vi "GetTextInformation.vi"(8 "error in (no error)":errorcluster, 10 "Input":string, 11 "Code128 in":refnum<class "Code128.lvclass">) -> (0 "error out":errorcluster, 1 "Text":string, 2 "Text Positions":T1[](array[typedef]), 3 "Code128 out":refnum<class "Code128.lvclass">)   [LabVIEW 2013, in "BarCodes.lvlib" / "Code128.lvclass"]
doc: "Returns an array of clusters describing how text will be sized and positioned and the actual text to place below the bar code. The Start Index is the index in the returned string that each text info entry refers to. The length is the number of characters in the returned string that each text info entry refers to. The Text Rectangle is the rectangle to draw text in. The Clearing Rectangle is the rectangle to paint with the barcode's light color to make the text clear and visible. The font information is passed into the text writing function."
uses:
  Code128.lvclass
  BarCode/TextPosition.ctl
  BarCodes.lvlib
  BarCode/BarCode.lvclass
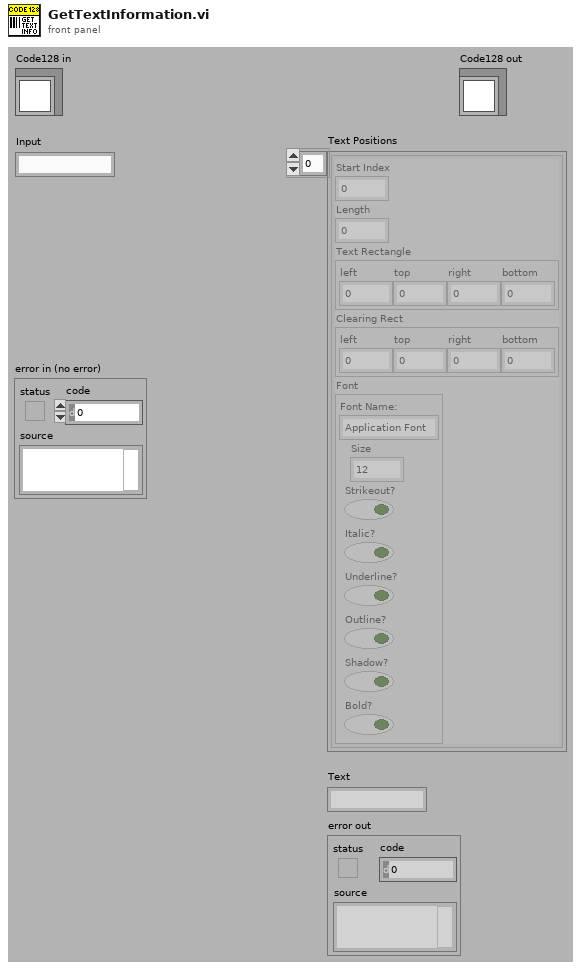
[diagram p1: front panel]
types:
  T1 = typedef "BarCodes.lvlib/BarCode.lvclass/TextPosition.ctl" = cluster{"Start Index":u8, "Length":u8, "Text Rectangle":cluster{"left":i16, "top":i16, "right":i16, "bottom":i16}, "Clearing Rect":cluster{"left":i16, "top":i16, "right":i16, "bottom":i16}, "Font":cluster{"Font Name:":string, "Size":i16, "Strikeout?":bool, "Italic?":bool, "Underline?":bool, "Outline?":bool, "Shadow?":bool, "Bold?":bool}}
  T2 = cluster{"left":i16, "top":i16, "right":i16, "bottom":i16}
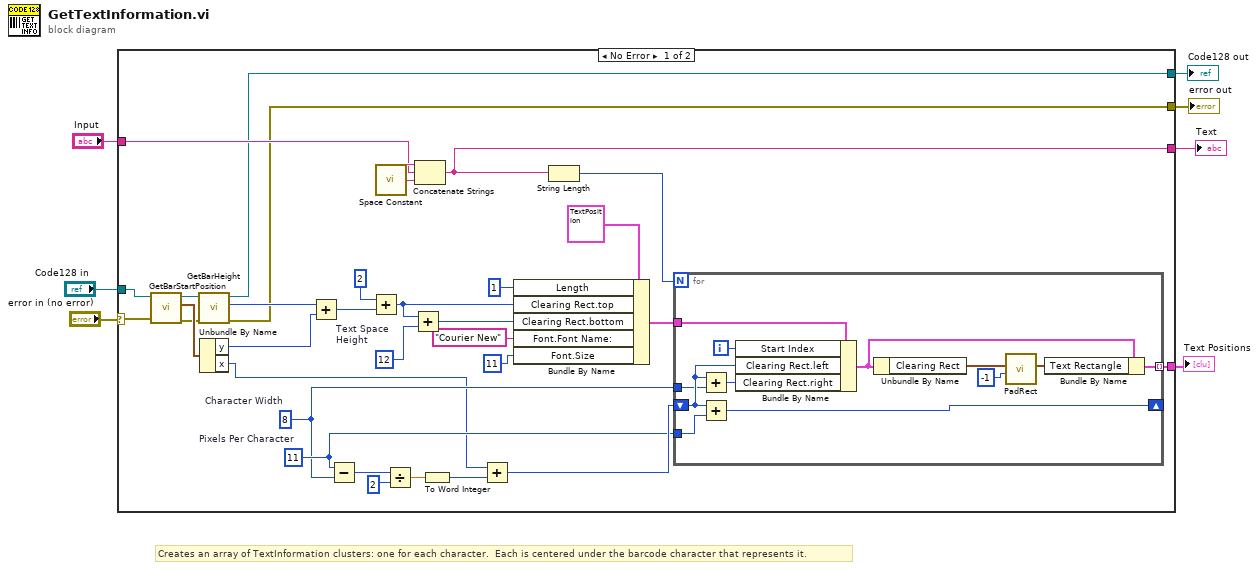
[diagram p0: block diagram]
diagram:
  # "Creates an array of TextInformation clusters: one for each character.  Each is centered under the barcode character that represents it."
  n1 = case shown="No Error" "error in (no error)" {
    selector: "error in (no error)" -> [w10 w52]
    tunnel: "Input" -> [w17 w54]
    tunnel: [w16 _] -> w6
    tunnel: [w15 w54] -> w5
    tunnel: "Code128 in" -> [w14 w53]
    tunnel: [w13 w53] -> w3
    tunnel: [w12 w52] -> w2
    frame No Error {
      w28 = i16 11  # Pixels Per Character
      w20 = i16 8  # Character Width
      w24 = i16 12  # Text Space Height
      n2 = call-dynamic "GetBarStartPosition.vi"("error in (no error)"=w10, "Code128 in"=w14) -> ("error out"=w37:errorcluster, "Start Position"=w39:cluster{"x":i16, "y":i16}, "Code128 out"=w38:refnum<class "Code128.lvclass">)  [unwired: 7 in]
      n3 = call-dynamic "GetBarHeight.vi"("error in (no error)"=w37, "Code128 in"=w38) -> ("error out"=w12:errorcluster, "Bar Height"=w36:u8, "Code128 out"=w13:refnum<class "Code128.lvclass">)  [unwired: 7 in]
      n4 = Unbundle By Name(w39) -> ("y"=w11:i16, "x"=w8:i16)
      n5 = Add(x=w36, y=w11) -> (x+y=w19:i16)
      n6 = Subtract(x=w28, y=w20) -> (x-y=w34:i16)
      n7 = Add(x=i16 2 ("y"), y=w19) -> (x+y=w18:i16)
      n8 = call <vilib>:"Space Constant.vi"() -> ("String"=w35:string)
      n9 = Divide(x=w34, y=i16 2) -> (x/y=w32:dbl)
      n10 = Add(x=w18, y=w24) -> (x+y=w23:i16)
      n11 = Concatenate Strings(w35, w17, w35) -> (w15:string)
      n12 = To Word Integer(number=w32) -> (16bit integer=w31:i16)
      n13 = Add(x=w8, y=w31) -> (x+y=w30:i16)
      n14 = Bundle By Name(cluster=T1 {"Start Index"=0, "Length"=0, "Text Rectangle"={"left"=0, "top"=0, "right"=0, "bottom"=0}, "Clearing Rect"={"left"=0, "top"=0, "right"=0, "bottom"=0}, "Font"={"Font Name:"="Application Font", "Size"=12, "Strikeout?"=FALSE, "Italic?"=FALSE, "Underline?"=FALSE, "Outline?"=FALSE, "Shadow?"=FALSE, "Bold?"=FALSE}} ("Text Position"), "Length"=u8 1, "Clearing Rect.top"=w18, "Clearing Rect.bottom"=w23, "Font.Font Name:"="Courier New", "Font.Size"=i16 11) -> (w21:T1)
      n15 = String Length(string=w15) -> (length=w29:i32)
      n16 = for {
        N: w29 -> [_]
        tunnel: w28 -> [w43]
        shift-right: [w41] -> _
        shift-left: w30 -> [w44]
        tunnel: w21 -> [w51]
        tunnel: [w46] -> w16 mode=indexing
        tunnel: w20 -> [w42]
        i -> [w40]
        n17 = Add(x=w44, y=w42) -> (x+y=w45:i16)
        n18 = Add(x=w44, y=w43) -> (x+y=w41:i16)
        n19 = Bundle By Name(cluster=w51, "Start Index"=w40, "Clearing Rect.left"=w44, "Clearing Rect.right"=w45) -> (w47:T1)
        n20 = Unbundle By Name(w47) -> ("Clearing Rect"=w50:T2)
        n21 = call "PadRect.vi"("Padding"=i8 -1, "Rectagle"=w50) -> ("Padded Rectangle"=w48:T2)  [unwired: 9 in]
        n22 = Bundle By Name(cluster=w47, "Text Rectangle"=w48) -> (w46:T1)
      }
    }
    frame Error {
    }
  }
  "error out" <- w2
  "Code128 out" <- w3
  "Text" <- w5
  "Text Positions" <- w6
